vi "계산기.vi"() -> ()   [LabVIEW 2018]
panel:
  out "Result":string
  in  "취소 버튼":bool
  in  "=":bool
  in  ".":bool
  in  "0":bool
  in  "+/-":bool
  in  "+":bool
  in  "3":bool
  in  "2":bool
  in  "1":bool
  in  "-":bool
  in  "6":bool
  in  "5":bool
  in  "4":bool
  in  "X":bool
  in  "9":bool
  in  "8":bool
  in  "7":bool
  in  "/":bool
  in  "x^(1/2)":bool
  in  "x^2":bool
  in  "1/x":bool
  in  "CLR":bool
  in  "C":bool
  in  "CE":bool
  in  "%":bool
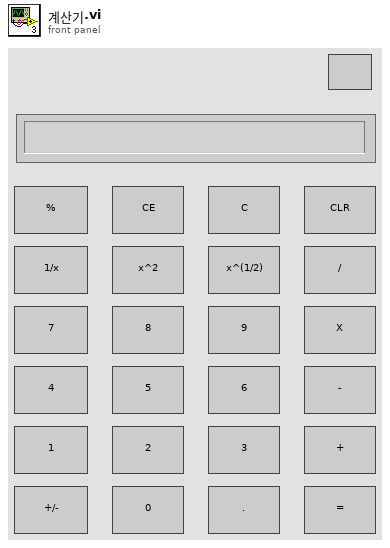
[diagram p1: front panel]
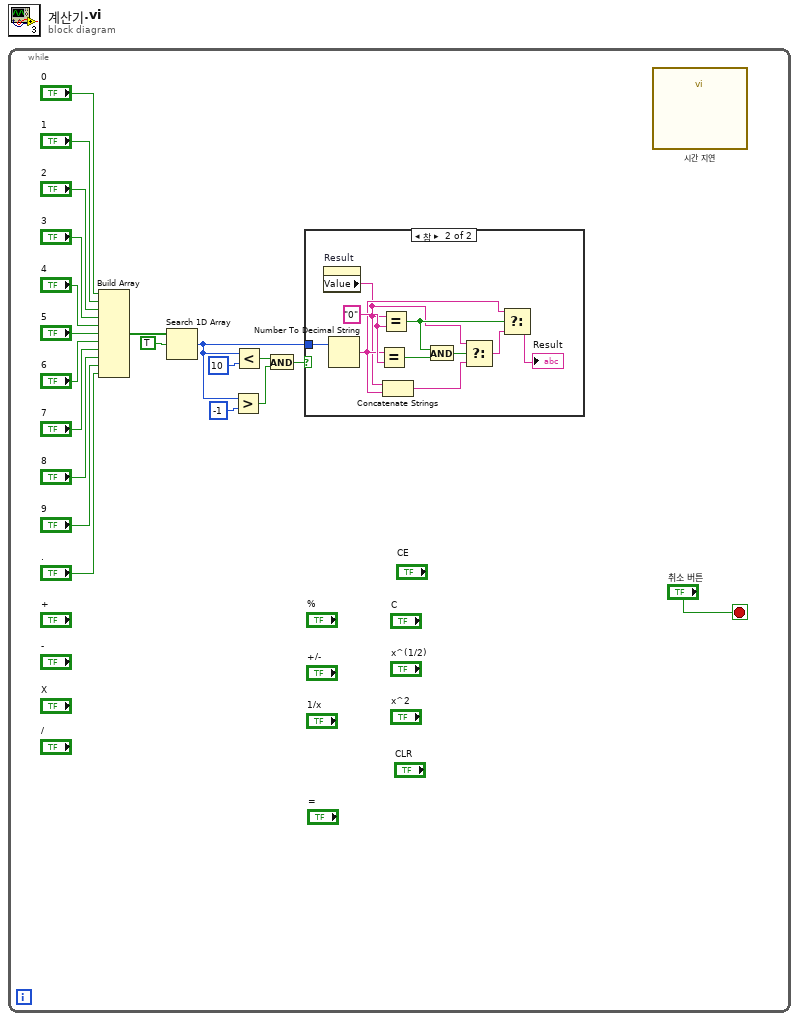
[diagram p0: block diagram]
diagram:
  n1 = while {
    stop <- "취소 버튼" stop-if-true
    n2 = Build Array("0", "1", "2", "3", "4", "5", "6", "7", "8", "9", ".") -> (w20:bool[])
    n3 = Search 1D Array(1D array=w20, element=TRUE) -> (index of element=w1:i32)  [unwired: 1 in]
    n4 = Greater?(x=w1, y=-1) -> (0:w4:bool)
    n5 = Less?(x=w1, y=10) -> (x < y?=w5:bool)
    n6 = And(x=w5, y=w4) -> (x .and. y?=w3:bool)
    n7 = case shown="참" w3 {
      tunnel: w1 -> [_ w30]
      frame False {
      }
      frame True {
        w24 = "0"
        n8 = property on="Result" class="Str"() -> ("Value"=w22:string)  [unwired: 2 in, 2 out]
        n9 = Number To Decimal String(number=w30) -> (decimal integer string=w23:string)  [unwired: 1 in]
        n10 = Equal?(x=w23, y=w24) -> (x = y?=w26:bool)
        n11 = Equal?(x=w22, y=w24) -> (x = y?=w25:bool)
        n12 = Concatenate Strings(w22, w23) -> (w29:string)
        n13 = And(x=w25, y=w26) -> (x .and. y?=w27:bool)
        n14 = Select(t=w22, s=w27, f=w29) -> (s? t:f=w28:string)
        n15 = Select(t=w23, s=w25, f=w28) -> (s? t:f=→"Result":string)
      }
    }
    n16 = call "시간 지연"() -> ()  [unwired: 11 in, 1 out]
  }
